vi "Agilent PSG MXG Series List Sweep.vi"() -> ()   [LabVIEW 2012]
doc: "This example shows how to configure a list sweep."
uses:
  <instrlib>/Agilent PSG MXG Series/Agilent PSG MXG Series.lvlib
panel:
  in  "VISA resource name":refnum<visa-resource-name>
  in  "Sweep Mode (3: Frequency and Power)":u16(ring)=3 items=["Off", "Frequency", "Power", "Frequency and Power"]
  in  "Power Array":dbl[](array[numeric])=[-20.0, -10.0, 0.0]
  in  "Frequency Array":dbl[](array[numeric])=[100000.0, 1000000.0, 10000000.0]
  in  "Dwell Time Array":dbl[](array[numeric])=[0.002, 0.002, 0.002]
  # "(c) 2012 National Instruments.  ALL RIGHTS RESERVED."
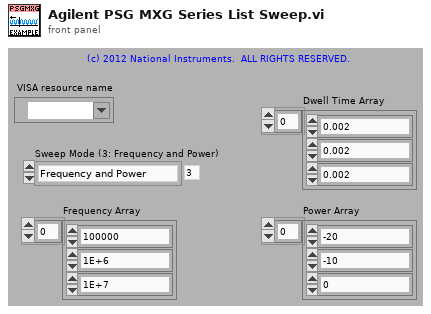
[diagram p1: front panel]
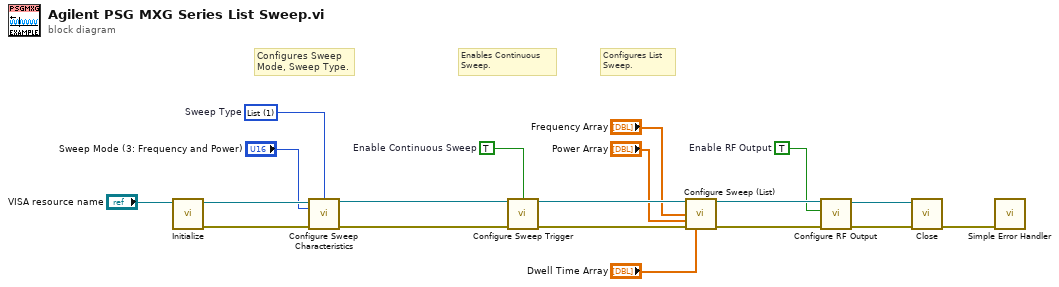
[diagram p0: block diagram]
diagram:
  w1 = TRUE  # Enable RF Output
  w13 = TRUE  # Enable Continuous Sweep
  w8 = u16 1 items=["Step", "List", "Ramp"]  # Sweep Type
  # "Configures List\nSweep."
  # "Enables Continuous\nSweep."
  # "Configures Sweep\nMode, Sweep Type."
  n1 = call <instrlib>:"Initialize.vi"("VISA resource name"="VISA resource name") -> ("error out"=w18:errorcluster, "VISA resource name out"=w19:refnum<visa-resource-name>)  [unwired: 3 in, 6 out]
  n2 = call <instrlib>:"Configure Sweep Characteristics.vi"("VISA resource name"=w19, "Sweep Type (0: Step)"=w8, "Sweep Mode (0: Off)"="Sweep Mode (3: Frequency and Power)", "error in (no error)"=w18) -> ("VISA resource name out"=w7:refnum<visa-resource-name>, "error out"=w6:errorcluster)  [unwired: 6 in, 4 out]
  n3 = call <instrlib>:"Configure Sweep Trigger.vi"("VISA resource name"=w7, "Enable Continuous Sweep (T:Enable)"=w13, "error in (no error)"=w6) -> ("VISA resource name out"=w16:refnum<visa-resource-name>, "error out"=w15:errorcluster)  [unwired: 5 in, 6 out]
  n4 = call <instrlib>:"Configure Sweep (List).vi"("VISA resource name"=w16, "Frequency Array"="Frequency Array", "Power Array"="Power Array", "error in (no error)"=w15, "Dwell Time Array"="Dwell Time Array") -> ("VISA resource name out"=w5:refnum<visa-resource-name>, "error out"=w4:errorcluster)  [unwired: 1 in, 8 out]
  n5 = call <instrlib>:"Configure RF Output.vi"("error in (no error)"=w4, "Enable RF Output (F:Disable)"=w1, "VISA resource name"=w5) -> ("error out"=w2:errorcluster, "VISA resource name out"=w3:refnum<visa-resource-name>)  [unwired: 4 in, 3 out]
  n6 = call <instrlib>:"Close.vi"("error in (no error)"=w2, "VISA resource name"=w3) -> ("error out"=w17:errorcluster)  [unwired: 9 out]
  n7 = call <vilib>:"Simple Error Handler.vi"("error in (no error)"=w17) -> ()  [unwired: 1 in, 8 out]
